vi "Limit Switch Control.vi"(11 "Run Mode":T1) -> (0 "Limit Switch 4":bool, 1 "Limit Switch 3":bool, 2 "Limit Switch 2":bool, 3 "Limit Switch 1":bool)   [LabVIEW 2014]
uses:
  SRE Enum.ctl
  Text Variable VIs/Read Number Variable.vi
  <vilib>/Rock Robotics/WPI/Switch/WPI_SwitchOpenLimit.vi
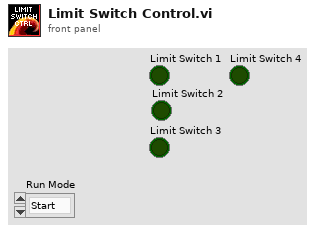
[diagram p1: front panel]
types:
  T1 = typedef "SRE Enum.ctl" = enum16{"Start", "Run", "End"}
  T2 = typedef "WPI_SwitchDevRef.ctl" = cluster{"DevStatus":errorcluster, "DIO Channel":T3, "Controller":T4, "CntIndex":T5, "Normally Closed":bool}
  T3 = typedef "FPGA_DIOChannel.ctl" = enum8{"DIO 0", "DIO 1", "DIO 2", "DIO 3", "DIO 4", "DIO 5", "DIO 6", "DIO 7", "DIO 8", "DIO 9", "DIO MXP 0", "DIO MXP 1", "DIO MXP 2", "DIO MXP 3", "DIO MXP 4", "DIO MXP 5", "DIO MXP 6", "DIO MXP 7", "DIO MXP 8", "DIO MXP 9", "DIO MXP 10", "DIO MXP 11", "DIO MXP 12", "DIO MXP 13", "DIO MXP 14", "DIO MXP 15", "Invalid"}
  T4 = typedef "FPGA_TypedefDigitalModule.ctl" = enum16{"Controller 1"}
  T5 = typedef "FPGA_CounterCtrSystemIndex.ctl" = enum8{"Ctr 0", "Ctr 1", "Ctr 2", "Ctr 3", "Ctr 4", "Ctr 5", "Ctr 6", "Ctr 7", "Invalid"}
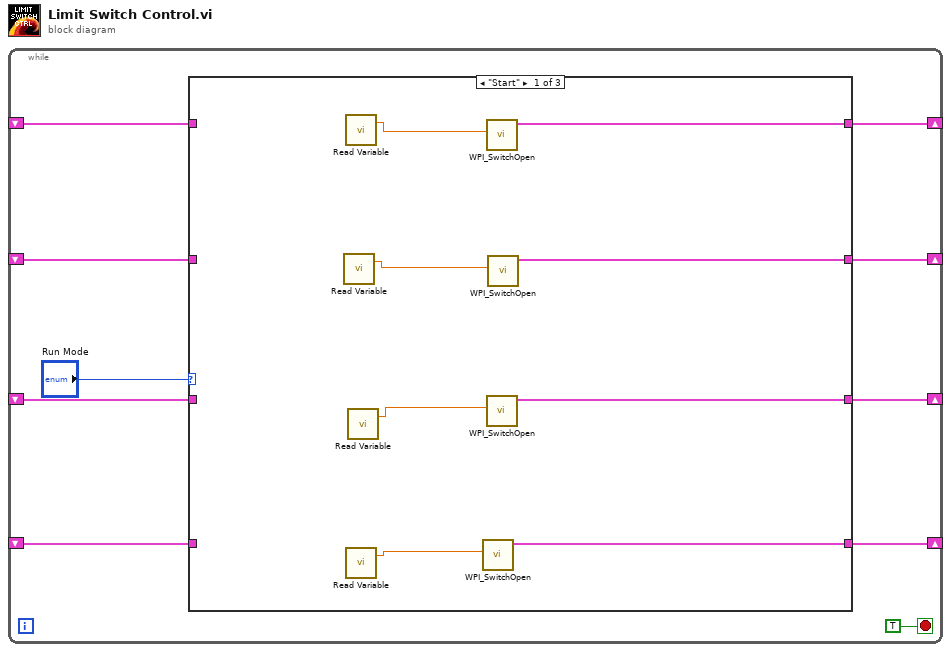
[diagram p0: block diagram]
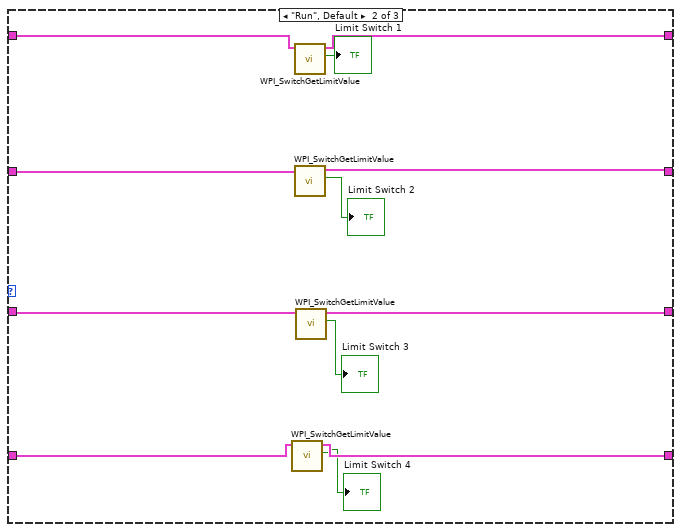
[diagram p2: hidden frame]
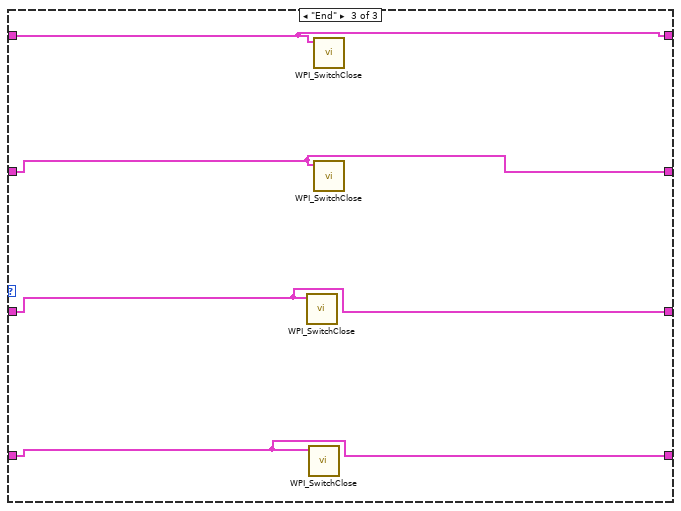
[diagram p3: hidden frame]
diagram:
  n1 = while {
    shift-right: [w7] -> _
    shift-left: _ -> [w4]
    shift-right: [w8] -> _
    shift-left: _ -> [w5]
    shift-right: [w9] -> _
    shift-left: _ -> [w3]
    shift-right: [w6] -> _
    shift-left: _ -> [w2]
    stop <- TRUE stop-if-true
    n2 = case shown="\"Start\"" "Run Mode" {
      tunnel: [w18 w26 w33] -> w9
      tunnel: [w17 w27 w32] -> w8
      tunnel: [w16 w29 w31] -> w7
      tunnel: [w15 w23 w34] -> w6
      tunnel: w5 -> [_ w28 w32]
      tunnel: w4 -> [_ w30 w31]
      tunnel: w3 -> [_ w25 w33]
      tunnel: w2 -> [_ w24 w34]
      frame "Start" {
        n3 = call-poly "Read Variable.vi"() -> ("number"=w11:dbl)  [unwired: 2 in, 1 out]
        n4 = call-poly "Read Variable.vi"() -> ("number"=w14:dbl)  [unwired: 2 in, 1 out]
        n5 = call-poly "Read Variable.vi"() -> ("number"=w12:dbl)  [unwired: 2 in, 1 out]
        n6 = call-poly "Read Variable.vi"() -> ("number"=w13:dbl)  [unwired: 2 in, 1 out]
        n7 = call-poly <vilib>:"WPI_SwitchOpen.vi"("DIO Channel"=w12) -> ("SwitchDevRef"=w15:T2)  [unwired: 9 in, 1 out]
        n8 = call-poly <vilib>:"WPI_SwitchOpen.vi"("DIO Channel"=w14) -> ("SwitchDevRef"=w16:T2)  [unwired: 9 in, 1 out]
        n9 = call-poly <vilib>:"WPI_SwitchOpen.vi"("DIO Channel"=w13) -> ("SwitchDevRef"=w18:T2)  [unwired: 9 in, 1 out]
        n10 = call-poly <vilib>:"WPI_SwitchOpen.vi"("DIO Channel"=w11) -> ("SwitchDevRef"=w17:T2)  [unwired: 9 in, 1 out]
      }
      frame "Run", Default {
        n11 = call <vilib>:"WPI_SwitchGetLimitValue.vi"("SwitchDevRef"=w24) -> ("Switch Pressed"=→"Limit Switch 4":bool, "SwitchDevRef"=w23:T2)  [unwired: 8 in, 1 out]
        n12 = call <vilib>:"WPI_SwitchGetLimitValue.vi"("SwitchDevRef"=w30) -> ("Switch Pressed"=→"Limit Switch 1":bool, "SwitchDevRef"=w29:T2)  [unwired: 8 in, 1 out]
        n13 = call <vilib>:"WPI_SwitchGetLimitValue.vi"("SwitchDevRef"=w28) -> ("Switch Pressed"=→"Limit Switch 2":bool, "SwitchDevRef"=w27:T2)  [unwired: 8 in, 1 out]
        n14 = call <vilib>:"WPI_SwitchGetLimitValue.vi"("SwitchDevRef"=w25) -> ("Switch Pressed"=→"Limit Switch 3":bool, "SwitchDevRef"=w26:T2)  [unwired: 8 in, 1 out]
      }
      frame "End" {
        n15 = call <vilib>:"WPI_SwitchClose.vi"("SwitchDevRef"=w33) -> ()  [unwired: 10 in, 1 out]
        n16 = call <vilib>:"WPI_SwitchClose.vi"("SwitchDevRef"=w34) -> ()  [unwired: 10 in, 1 out]
        n17 = call <vilib>:"WPI_SwitchClose.vi"("SwitchDevRef"=w31) -> ()  [unwired: 10 in, 1 out]
        n18 = call <vilib>:"WPI_SwitchClose.vi"("SwitchDevRef"=w32) -> ()  [unwired: 10 in, 1 out]
      }
    }
  }
